vi "Configure DAQ (by ref).vi"(0 "System Ref":tag, 1 "Cal Files Path":path, 4 "Config":T3={"DAQ Settings"={"Trigger Type"=enum."Manual", "Trigger Samples"=0, "Pretrigger Samples"=0, "Trigger Interval"=0.0, "Time Units"=FALSE, "Auto Save"=FALSE, "Sample Rate"=7.0, "Select Analog"=FALSE, "Trigger Value"=0.0, "Trigger Stop Method"=enum."Use Samples Value to Stop Trigger", "Rate Sec/Min"=FALSE, "Save Mode"=enum."Single File", "File Size Limit"=0.0, "Log File Type"=enum."Basic", "Trigger Data Index"=0, "Log Rate"=7.0, "Rate Sec/Min (Log)"=FALSE, "Sample Rate (S/s)"=0.0, "Log Rate (S/s)"=0.0}, "Channels"=[], "Header"={"CA Number"="", "Test Name"="", "Serial Number"="", "Technician"=""}, "Graph Settings"={"Graph Labels"=[], [], [], [], [], [], [], [], [], [], [], [], [], "Graph Toggles"=[], "Axis Toggles"=[], "Graph Range"=enum."1"}, "Test Limits"=[], "All Type Info"=[], "Save Mode"=enum."Single File", "Data Base Path"=path ""} {"DAQ Settings"."Trigger Interval" min=0.0; "DAQ Settings"."Pretrigger Samples" min=0; "DAQ Settings"."Trigger Samples" min=0}, 5 "Channel Filter":bool[](array[boolean])=[FALSE, TRUE, TRUE, TRUE, TRUE, TRUE, TRUE, TRUE, TRUE, TRUE, TRUE, TRUE, TRUE, TRUE, TRUE, TRUE, TRUE, TRUE, TRUE, TRUE, TRUE, TRUE, TRUE, TRUE, TRUE, TRUE, TRUE, TRUE, TRUE, TRUE, TRUE, TRUE, TRUE, TRUE, TRUE, TRUE, TRUE, TRUE, TRUE, TRUE, TRUE, TRUE, TRUE, TRUE, TRUE, TRUE, TRUE, TRUE, TRUE], 7 "Sensor (scaling)":T2(array[cluster]), 8 "Manual/Timed Trigger":bool, 9 "Mode":enum16{"Init", "Acquire", "Clear"}(ring), 11 "System Type":T1, 14 "Total Channel Count":i16, 15 "Time Offset":dbl) -> (16 "Pretrigger Size":i32, 20 "Input Task OUT":refnum<k21>, 21 "Acquiring Data":bool, 22 "Ctr Task OUT":refnum<k21>, 24 "DAQ Complete Trigger":bool, 25 "Data":sgl[][](array[numeric]), 26 "DI Task OUT":refnum<k21>, 27 "error out":errorcluster={"status"=TRUE, "code"=-10621, "source"="AI Control"})   [LabVIEW 2023]
uses:
  Type Defs and Controls/Sensor Config.ctl
  Type Defs and Controls/DAQ Settings.ctl
  Type Defs and Controls/Trigger Stop Method.ctl
  Type Defs and Controls/Log File Type.ctl
  Type Defs and Controls/Channel Config.ctl
  Type Defs and Controls/Header.ctl
  Type Defs and Controls/Graph Settings Type Def.ctl
  Type Defs and Controls/Test Limits.ctl
  Type Defs and Controls/All Part Info.ctl
  Type Defs and Controls/Part Info.ctl
  Type Defs and Controls/System Type.ctl
  Type Defs and Controls/Coeffs Cluster Type Def.ctl
  <vilib>/DAQmx/read.llb/DAQmx Read (Counter 1D DBL 1Chan NSamp).vi
  <vilib>/DAQmx/read.llb/DAQmx Read (Analog 2D DBL NChan NSamp).vi
  <vilib>/DAQmx/miscellaneous.llb/DAQmx Fill In Error Info.vi
  <vilib>/measure/mamon.llb/Trigger Detection for 1 Channel (obs).vi
  <vilib>/measure/NI_MAPro.lvlib
  <resource>/objmgr/daqmx.rc
panel:
  out "Acquiring Data":bool
  # "EGU"
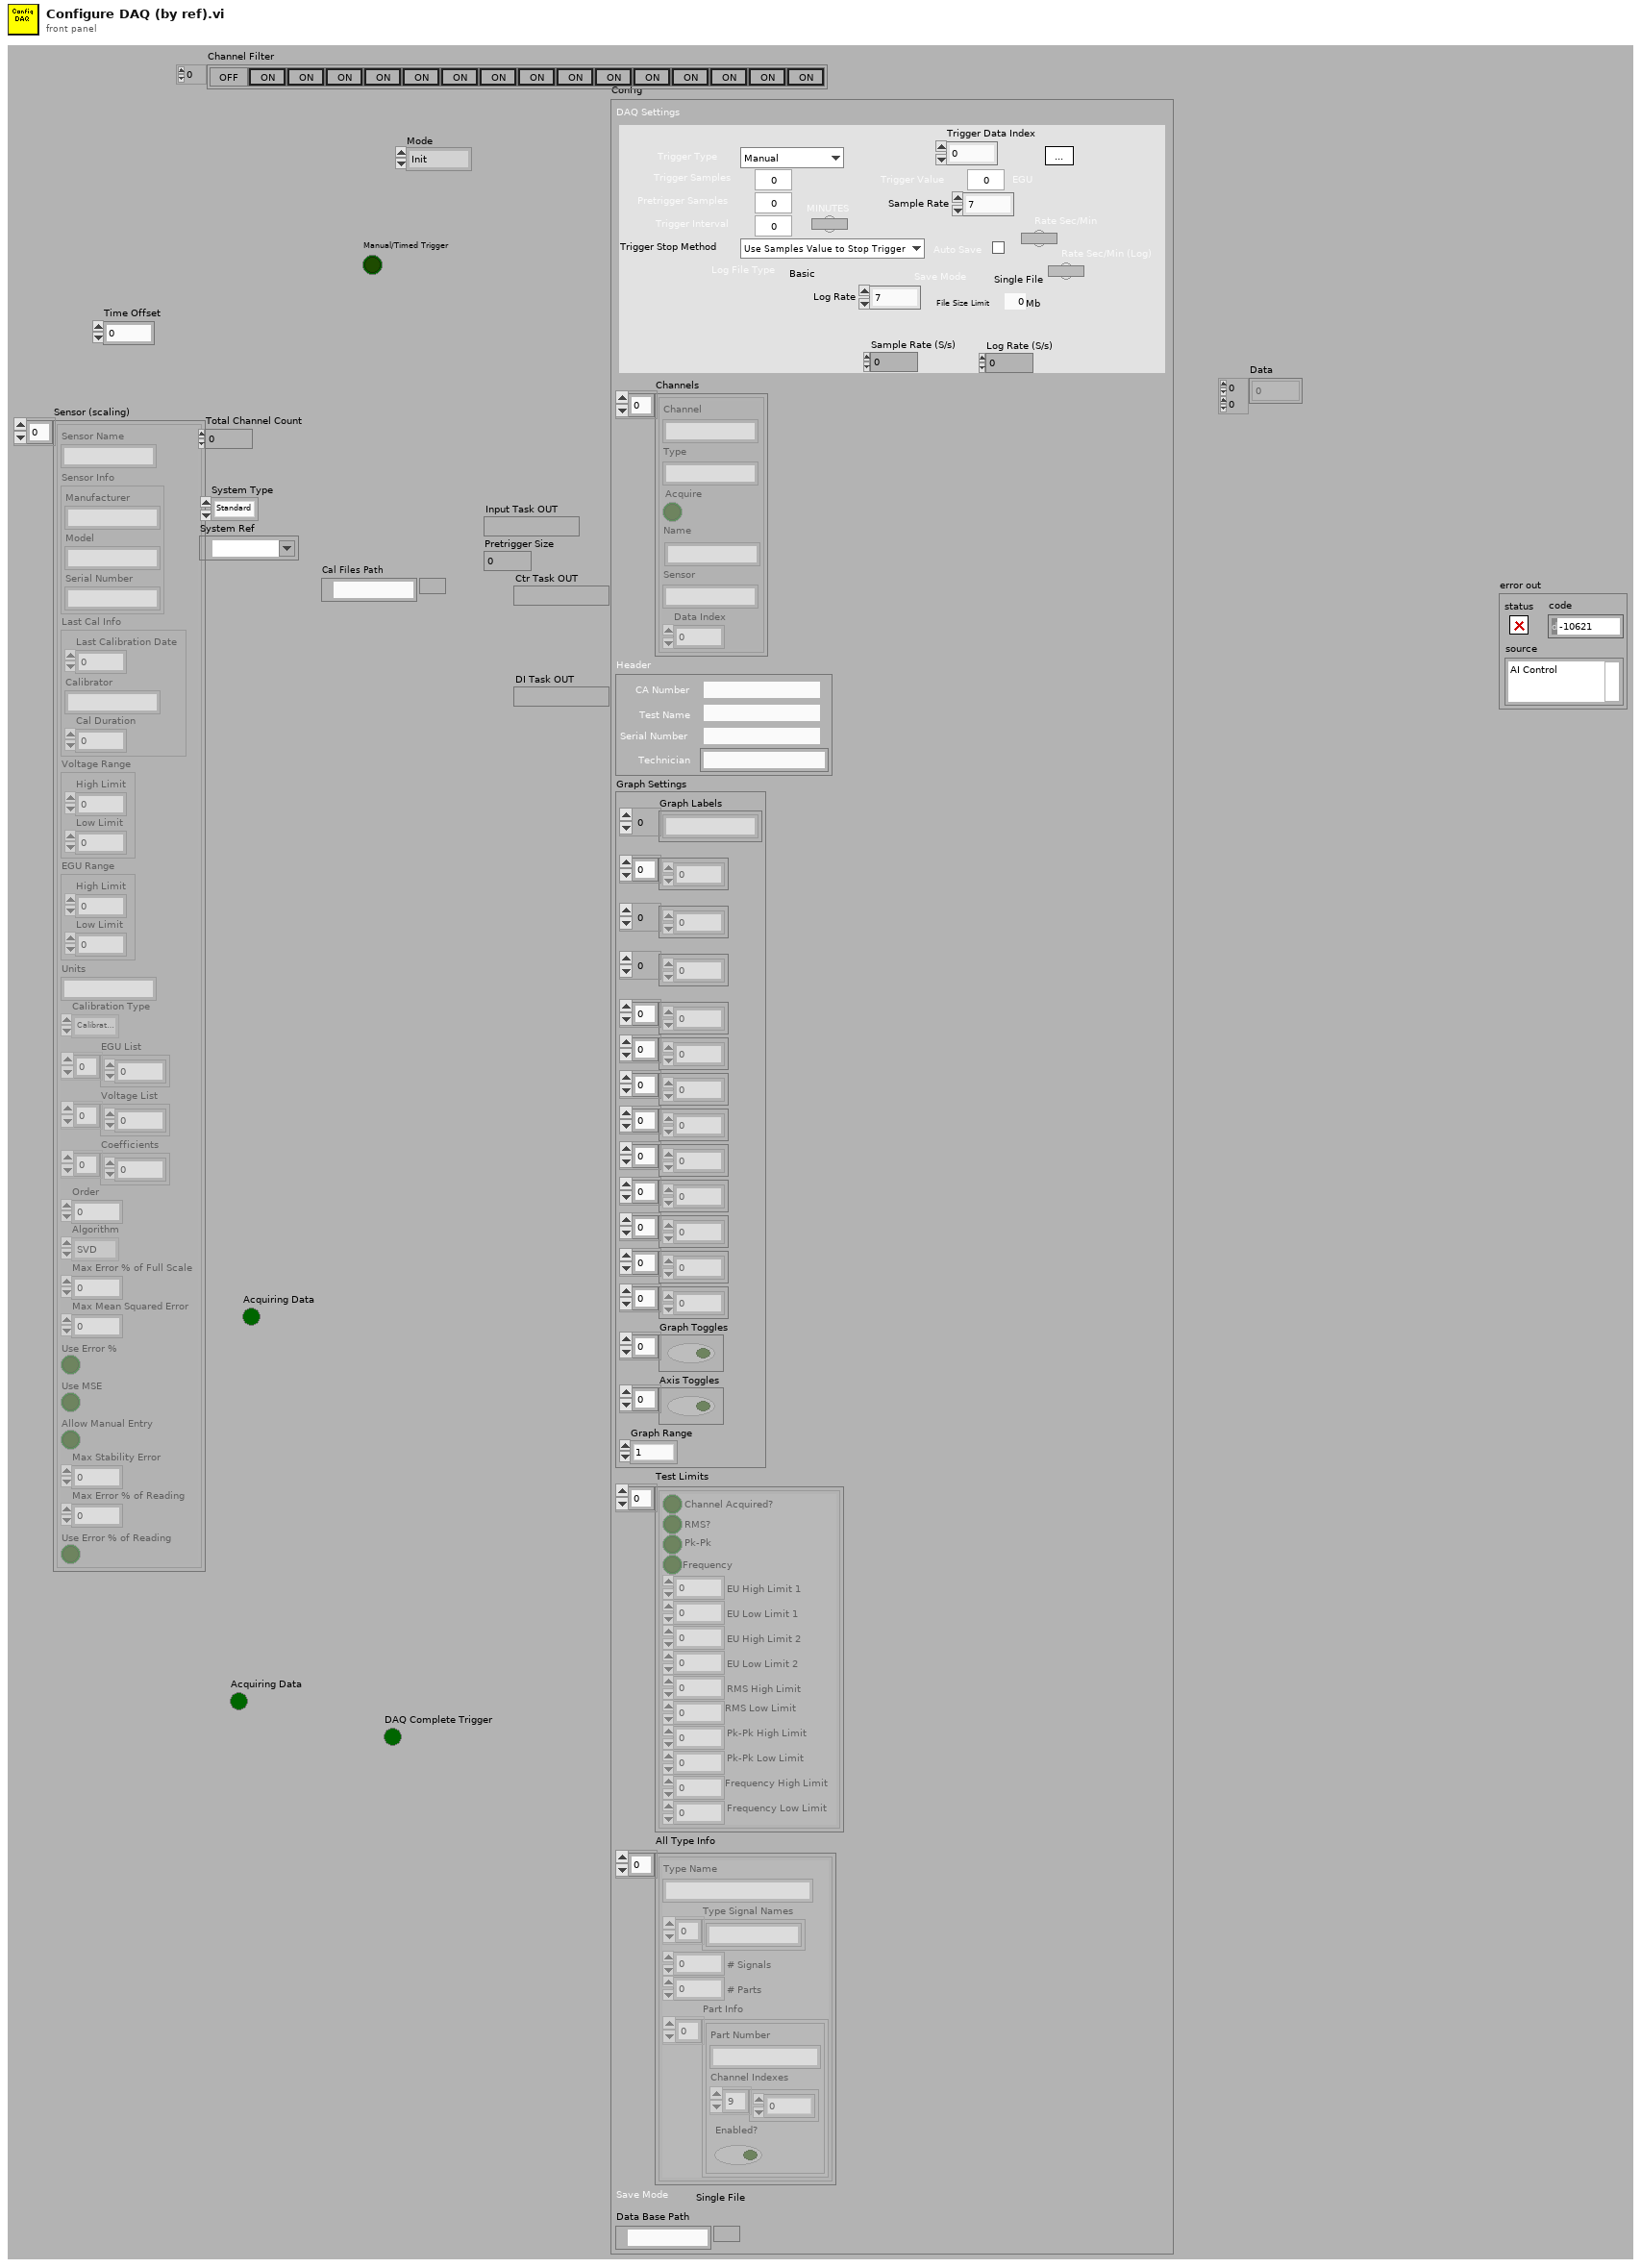
[diagram p1: front panel]
types:
  T1 = typedef "System Type.ctl" = enum16{"Standard", "Deformation", "Standard 8TC"}
  T2 = cluster{"Sensor Name":string, "Sensor Info":cluster{"Manufacturer":string, "Model":string, "Serial Number":string}, "Last Cal Info":cluster{"Last Calibration Date":dbl, "Calibrator":string, "Cal Duration":i32}, "Voltage Range":cluster{"High Limit":dbl, "Low Limit":dbl}, "EGU Range":cluster{"High Limit":dbl, "Low Limit":dbl}, "Units":string, "Calibration Type":enum16{"Calibrate Analog", "Compare Analog Calibration"}, "EGU List":dbl[], "Voltage List":dbl[], "Coefficients":dbl[], "Order":i32, "Algorithm":enum32{"SVD", "Givens", "Givens2", "Householder", "LU Decomposition", "Cholesky"}, "Max Error % of Full Scale":dbl, "Max Mean Squared Error":dbl, "Use Error %":bool, "Use MSE":bool, "Allow Manual Entry":bool, "Max Stability Error":dbl, "Max Error % of Reading":dbl, "Use Error % of Reading":bool}[]
  T3 = typedef "Sensor Config.ctl" = cluster{"DAQ Settings":T4, "Channels":T7[], "Header":T8, "Graph Settings":T9, "Test Limits":T10[], "All Type Info":T11, "Save Mode":enum16{"Single File", "Segmented Files", "New File at Midnight"}, "Data Base Path":path}
  T4 = typedef "DAQ Settings.ctl" = cluster{"Trigger Type":enum16{"Manual", "Timed", "Analog Rising", "Analog Falling"}, "Trigger Samples":i32, "Pretrigger Samples":i32, "Trigger Interval":dbl, "Time Units":bool, "Auto Save":bool, "Sample Rate":dbl, "Select Analog":bool, "Trigger Value":dbl, "Trigger Stop Method":T5, "Rate Sec/Min":bool, "Save Mode":enum16{"Single File", "Segmented Files", "New File at Midnight"}, "File Size Limit":dbl, "Log File Type":T6, "Trigger Data Index":u32, "Log Rate":dbl, "Rate Sec/Min (Log)":bool, "Sample Rate (S/s)":dbl, "Log Rate (S/s)":dbl}
  T5 = typedef "Trigger Stop Method.ctl" = enum16{"Use Samples Value to Stop Trigger", "Use Threshold to Stop Trigger"}
  T6 = typedef "Log File Type.ctl" = enum16{"Basic", "RTS"}
  T7 = typedef "Channel Config.ctl" = cluster{"Channel":string, "Type":string, "Acquire":bool, "Name":string, "Sensor":string, "Data Index":u32}
  T8 = typedef "Header.ctl" = cluster{"CA Number":string, "Test Name":string, "Serial Number":string, "Technician":string}
  T9 = typedef "Graph Settings Type Def.ctl" = cluster{"Graph Labels":string[], u8[], i16[], u32[], u8[], u8[], u8[], u32[], u8[], u8[], u8[], dbl[], dbl[], "Graph Toggles":bool[], "Axis Toggles":bool[], "Graph Range":enum16{"1", "2", "3", "4", "5", "10", "15", "30", "60"}}
  T10 = typedef "Test Limits.ctl" = cluster{"Channel Acquired?":bool, "RMS?":bool, "Pk-Pk":bool, "Frequency":bool, "EU High Limit 1":dbl, "EU Low Limit 1":dbl, "EU High Limit 2":dbl, "EU Low Limit 2":dbl, "RMS High Limit":dbl, "RMS Low Limit":dbl, "Pk-Pk High Limit ":dbl, "Pk-Pk Low Limit":dbl, "Frequency High Limit":dbl, "Frequency Low Limit":dbl}
  T11 = typedef "All Part Info.ctl" = cluster{"Type Name":string, "Type Signal Names":string[], "# Signals":i32, "# Parts":i32, "Part Info":T12[]}[]
  T12 = typedef "Part Info.ctl" = cluster{"Part Number":string, "Channel Indexes":u16[], "Enabled?":bool}
  T13 = typedef "Coeffs Cluster Type Def.ctl" = cluster{"AI Coeffs":cluster{"Coefficients":dbl[]}[]}
  T14 = cluster{"Coefficients":cluster{"Coefficients":dbl[]}[]}
  T15 = enum16{"Manual", "Timed", "Analog Rising", "Analog Falling"}
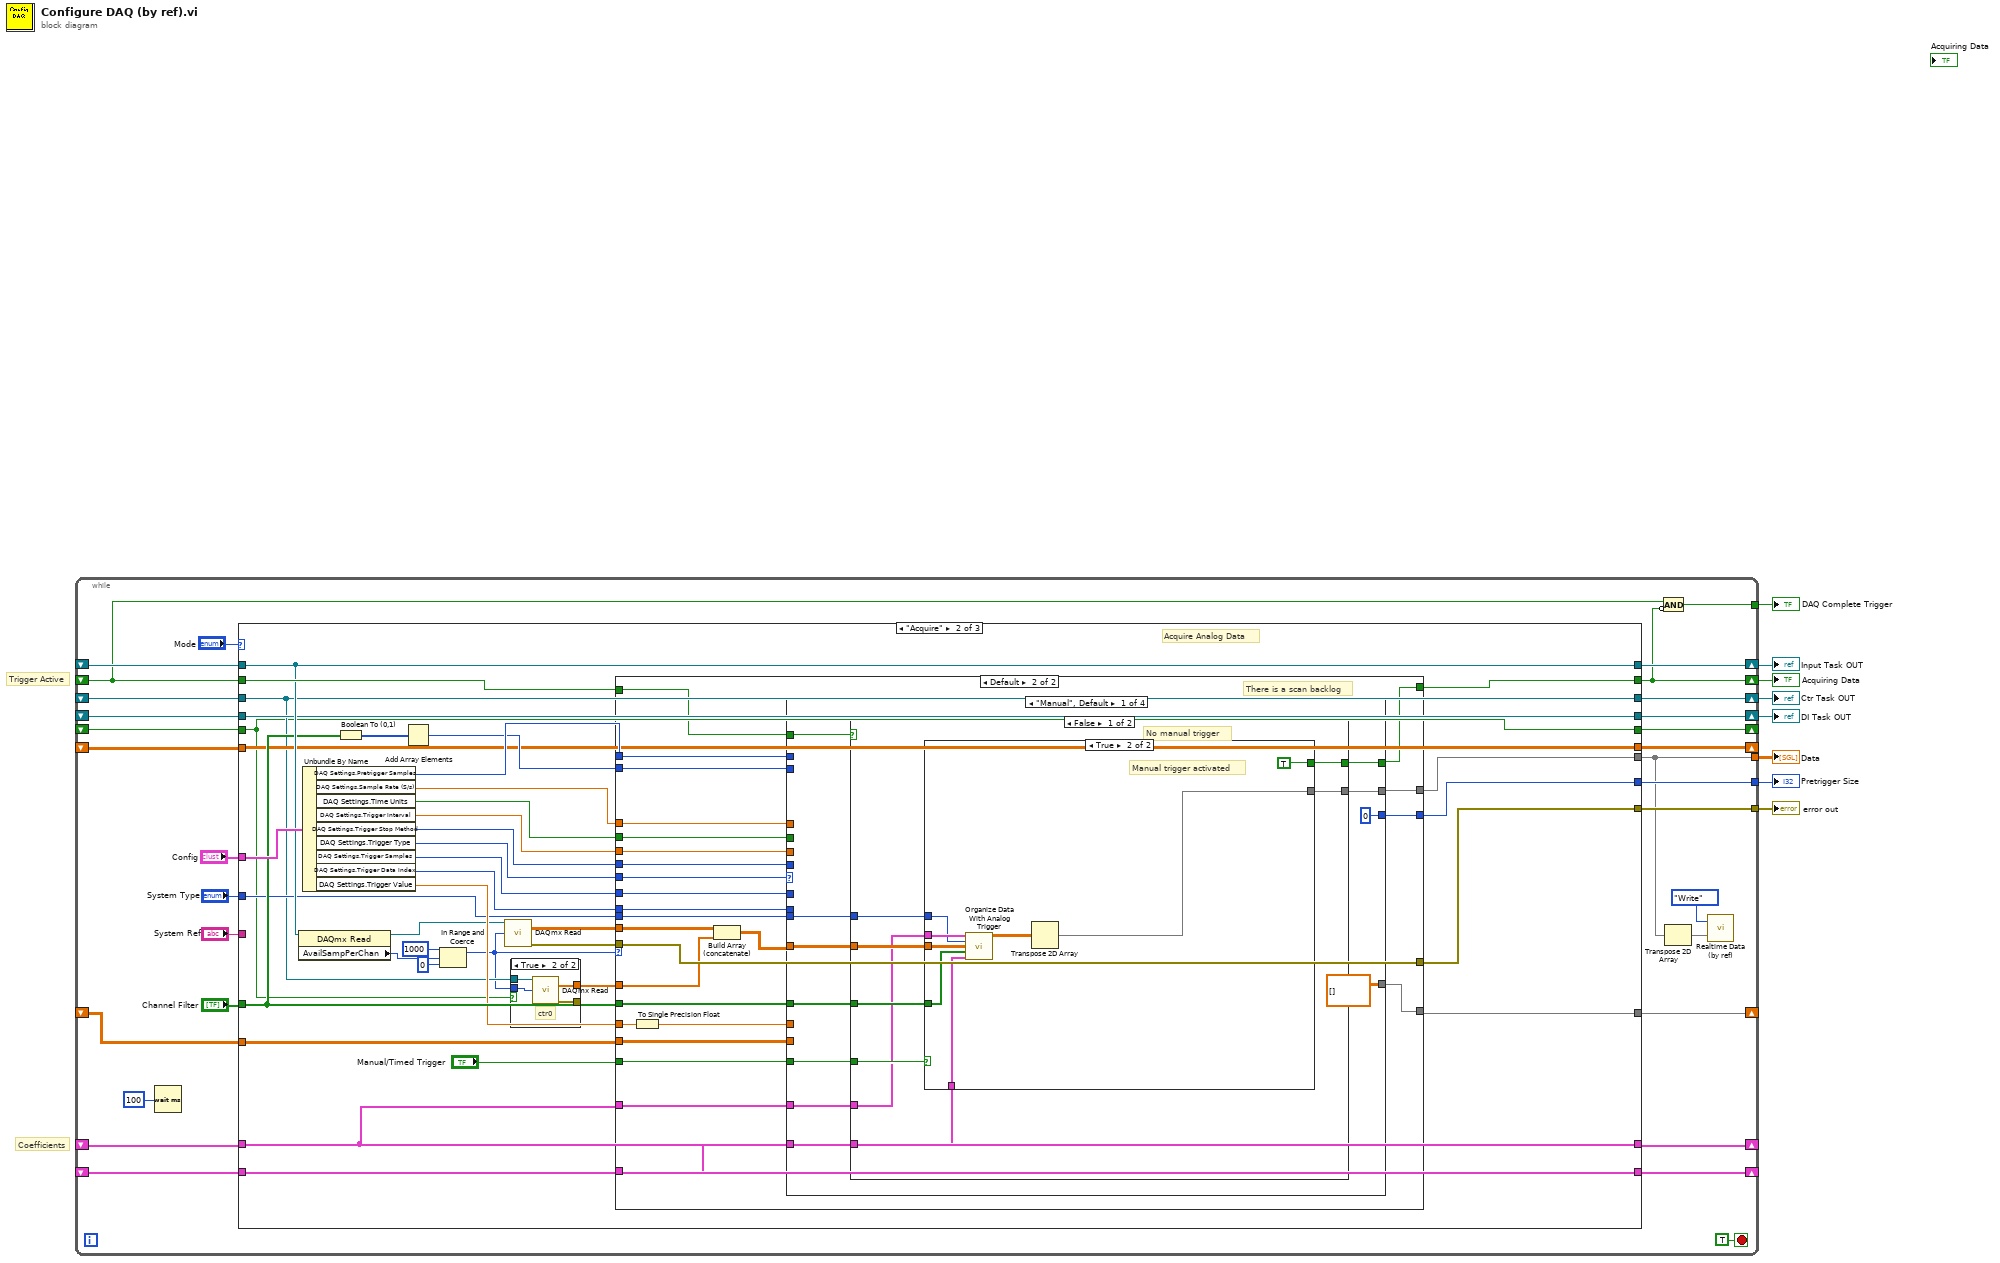
[diagram p0: block diagram]
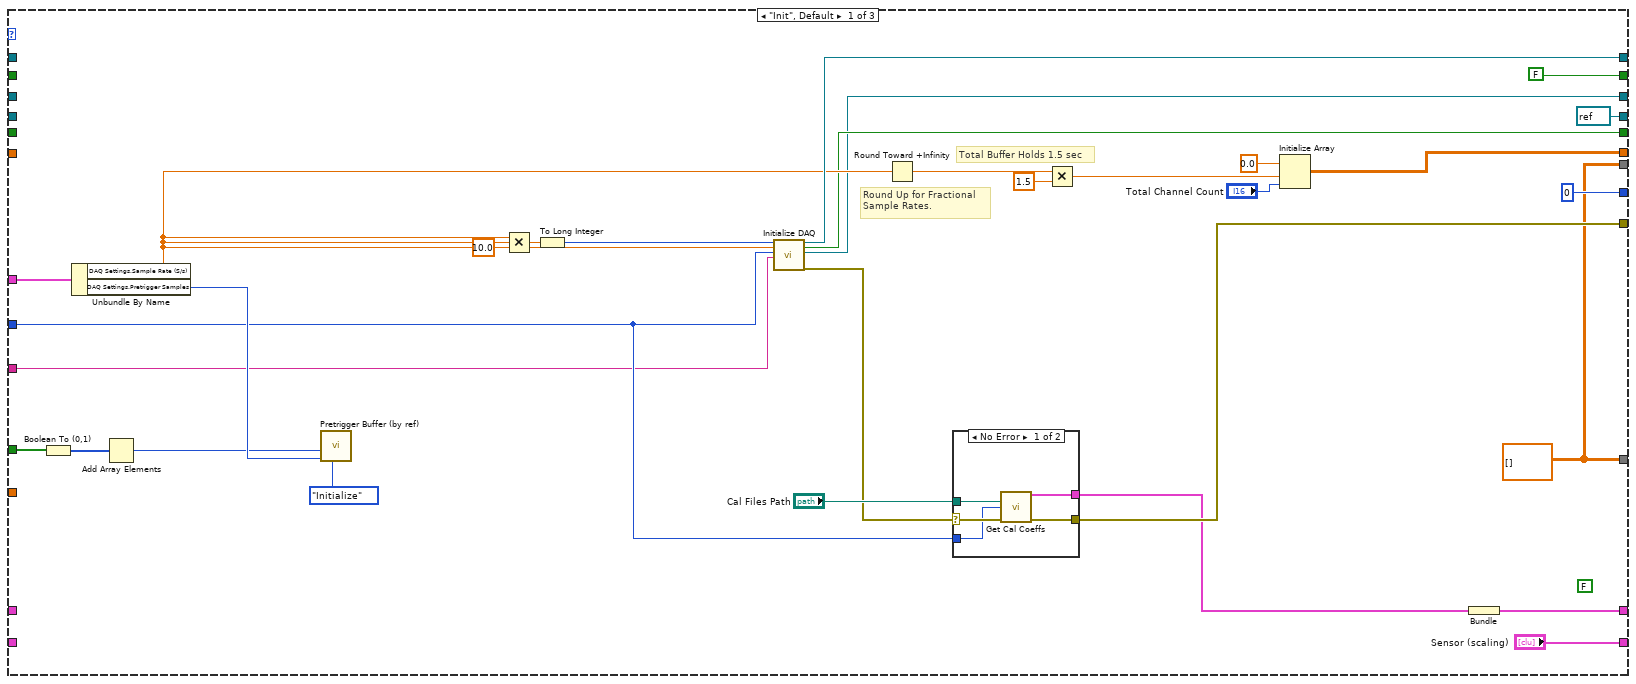
[diagram p2: hidden frame]
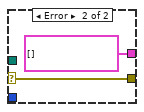
[diagram p3: hidden frame]
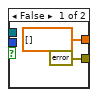
[diagram p4: hidden frame]
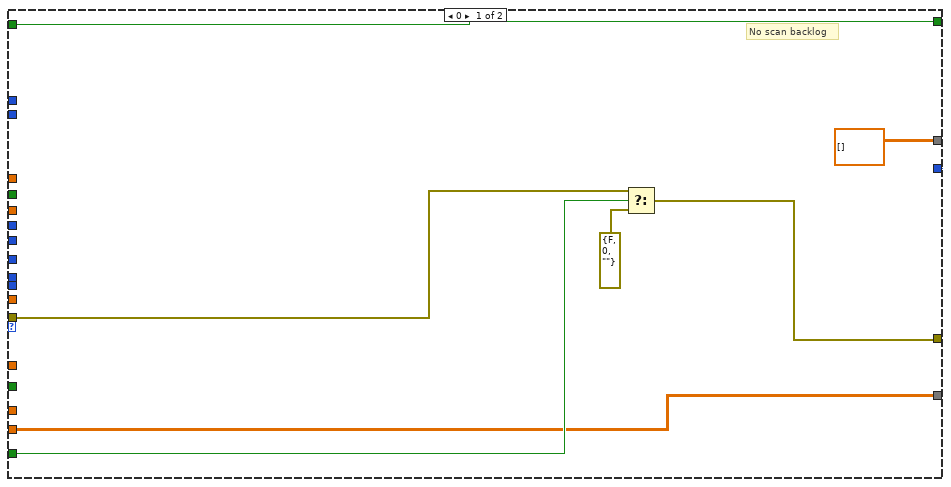
[diagram p5: hidden frame]
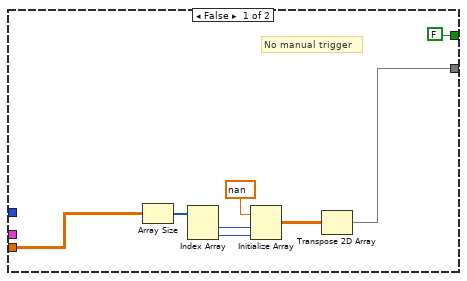
[diagram p6: hidden frame]
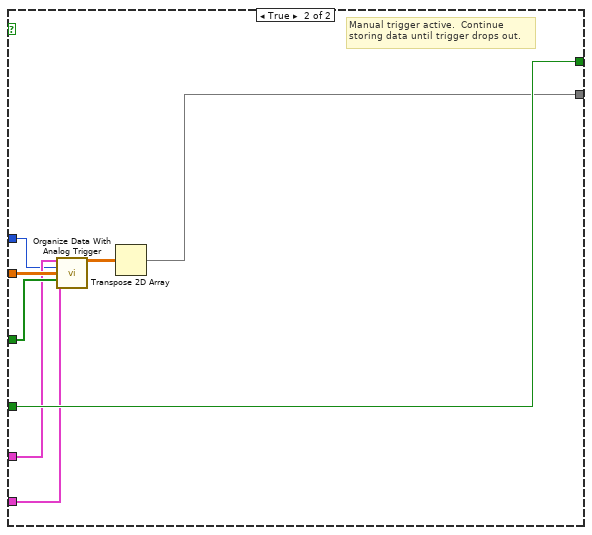
[diagram p7: hidden frame]
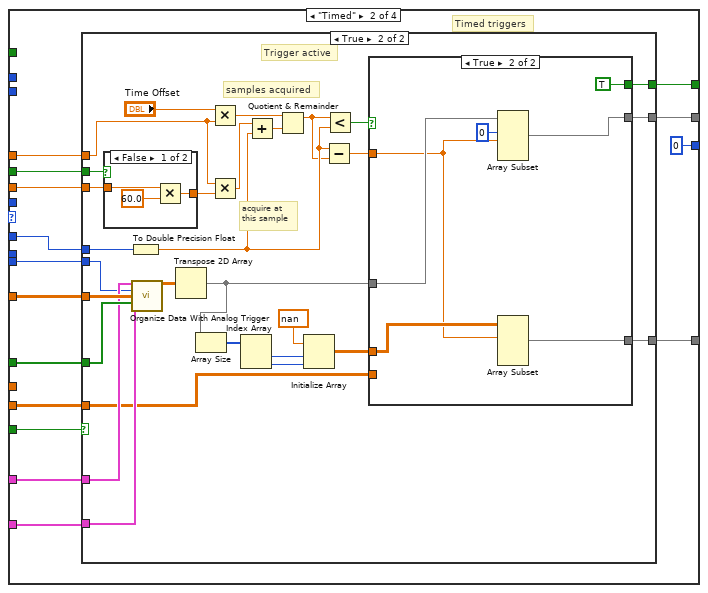
[diagram p8: hidden frame]
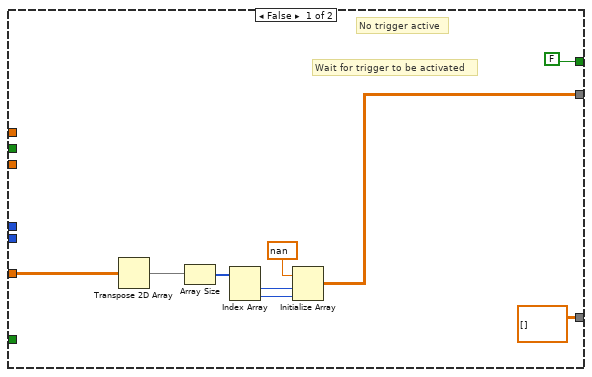
[diagram p9: hidden frame]
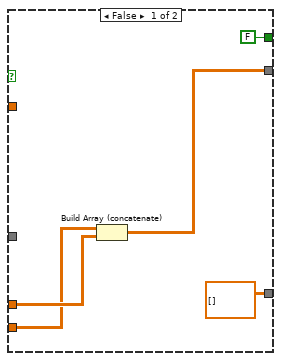
[diagram p10: hidden frame]
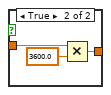
[diagram p11: hidden frame]
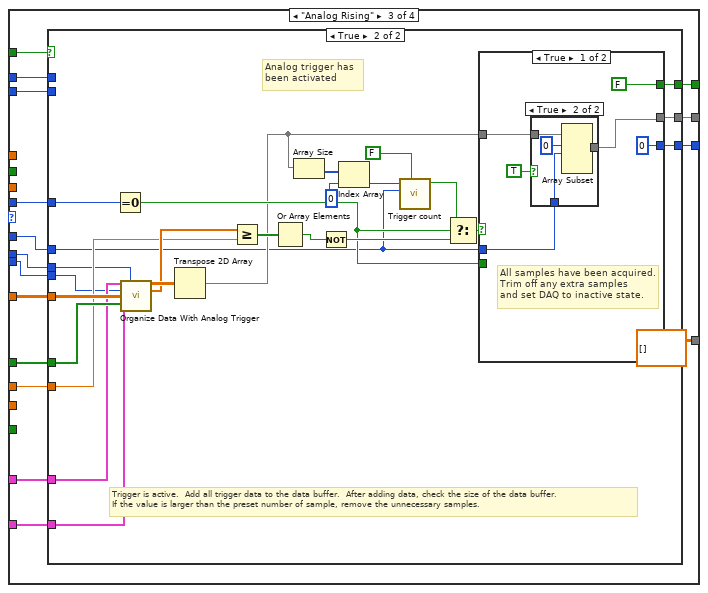
[diagram p12: hidden frame]
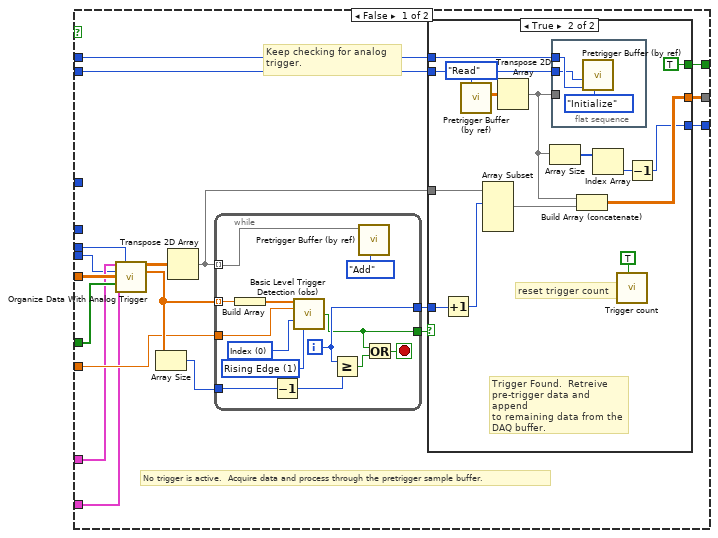
[diagram p13: hidden frame]
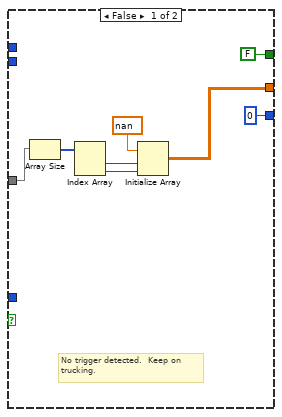
[diagram p14: hidden frame]
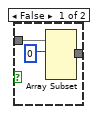
[diagram p15: hidden frame]
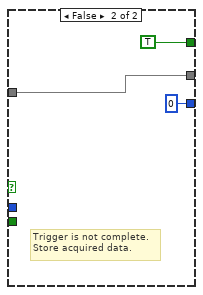
[diagram p16: hidden frame]
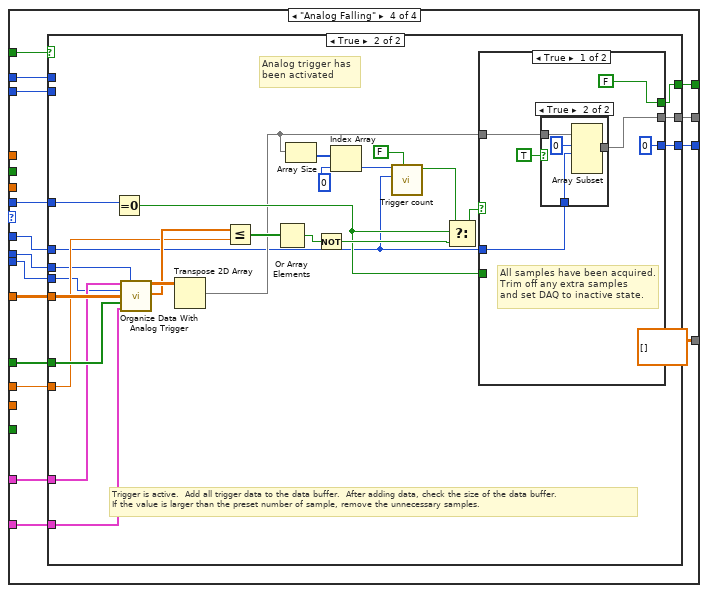
[diagram p17: hidden frame]
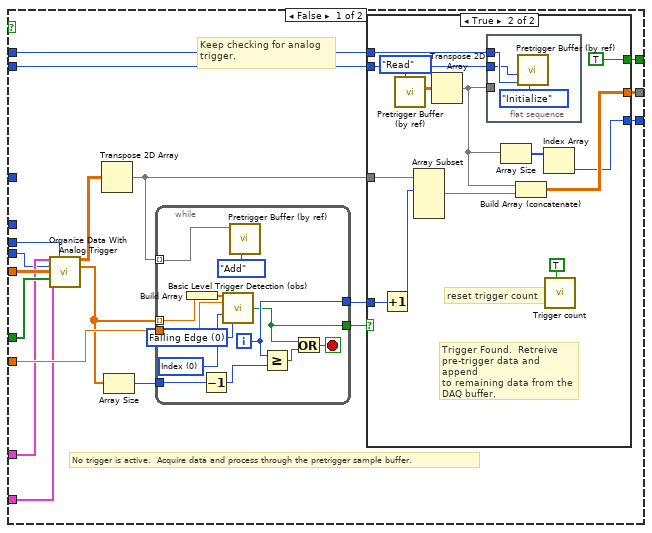
[diagram p18: hidden frame]
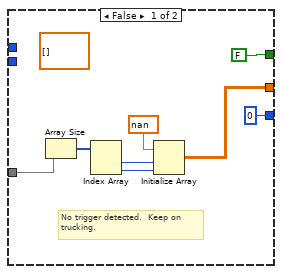
[diagram p19: hidden frame]
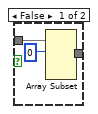
[diagram p20: hidden frame]
diagram:
  # "Coefficients"
  # "Trigger Active"
  n1 = while {
    shift-right: [w34] -> w5
    shift-left: _ -> [w36]
    tunnel: [w37] -> w8
    shift-right: [w32] -> w7
    shift-left: _ -> [w30]
    tunnel: [w31] -> w6
    shift-right: [w29] -> _
    shift-left: _ -> [w28]
    shift-right: [w24] -> _
    shift-left: _ -> [w25]
    tunnel: [w23] -> w4
    shift-right: [w22] -> _
    shift-left: _ -> [w21]
    shift-right: [w18] -> _
    shift-left: _ -> [w19]
    tunnel: [w17] -> w3
    shift-right: [w16] -> w2
    shift-left: _ -> [w15]
    shift-right: [w14] -> w1
    shift-left: _ -> [w13]
    shift-right: [w11] -> _
    shift-left: _ -> [w10]
    stop <- TRUE stop-if-true
    n2 = Wait (ms)(milliseconds to wait=u32 100) -> ()  [unwired: 1 out]
    n3 = case shown="\"Acquire\"" "Mode" {
      tunnel: [w56 w91 errorcluster {"status"=FALSE, "code"=0, "source"=""} ("error out")] -> w37
      tunnel: w36 -> [_ w104 w505]
      tunnel: "Config" -> [w68 w108 _]
      tunnel: [w60 w104 refnum<k21> refnum ("task out")] -> w34
      tunnel: [FALSE w112 FALSE] -> w32
      tunnel: w30 -> [_ w110 _]
      tunnel: [w48 w88 w501] -> w17
      tunnel: "Channel Filter" -> [w58 w101 _]
      tunnel: ["Sensor (scaling)" w107 w507] -> w29
      tunnel: w28 -> [_ w107 w507]
      tunnel: [w45 w93 T13 {"AI Coeffs"=[]} ("Coefficients")] -> w24
      tunnel: w25 -> [_ w93 _]
      tunnel: [0 w99 0] -> w23
      tunnel: [w48 w96 w501] -> w22
      tunnel: w21 -> [_ w95 _]
      tunnel: w19 -> [_ w89 w502]
      tunnel: [w49 w89 w502] -> w18
      tunnel: [w41 w80 refnum<k21> refnum ("DO Task OUT")] -> w16
      tunnel: w15 -> [_ w80 w499]
      tunnel: [refnum<k21> refnum ("DO Task OUT") w92 refnum<k21> refnum ("DO Task OUT")] -> w14
      tunnel: w13 -> [_ w92 w497]
      tunnel: "System Type" -> [w43 w81 _]
      tunnel: [w42 w78 FALSE ("Ctr Present")] -> w11
      tunnel: w10 -> [_ w78 _]
      tunnel: "System Ref" -> [w40 _ _]
      frame "Init", Default {
        (unwired) FALSE ("data")
        w48 = sgl[][] []
        # "Round Up for Fractional\nSample Rates."
        # "Total Buffer Holds 1.5 sec"
        n4 = Boolean To (0,1)(Boolean=w58) -> (0, 1=w64:i16[])
        n5 = Unbundle By Name(w68) -> ("DAQ Settings.Sample Rate (S/s)"=w53:dbl, "DAQ Settings.Pretrigger Samples"=w65:i32)
        n6 = Add Array Elements(numeric array=w64) -> (sum=w63:i16)
        n7 = call "Pretrigger Buffer (by ref).vi"("Mode"=enum16{"Initialize", "Add", "Read"}."Initialize", "Pretrigger Length"=w65, "# Channels"=w63) -> ()  [unwired: 6 in, 2 out]
        n8 = Multiply(x=w53, y=sgl 10.0) -> ()  [unwired: 1 out]
        n9 = To Long Integer(number=w53) -> (32bit integer=w61:i32)
        n10 = call "Initialize DAQ.vi"("number of samples"=w61, "rate"=w53, "System Type"=w43, "System Ref"=w40) -> ("AI Task OUT"=w60:refnum<k21>, "Ctr Present"=w42:bool, "Ctr Task OUT"=w41:refnum<k21>, "error out"=w57:errorcluster)  [unwired: 12 in]
        n11 = Round Toward +Infinity(x=w53) -> (ceil(x): smallest int >= x=w47:dbl)
        n12 = case shown="No Error" w57 {
          selector: w57 -> [w72 w76]
          tunnel: "Cal Files Path" -> [w74 _]
          tunnel: [w73 cluster{"Coefficients":dbl[]}[] [] ("Coefficients")] -> w46
          tunnel: [w71 w76] -> w56
          tunnel: w43 -> [w70 _]
          frame No Error {
            n13 = call "Get Cal Coeffs.vi"("Cal Files Path"=w74, "System Type"=w70, "Error IN"=w72) -> ("AI Coeffs"=w73:cluster{"Coefficients":dbl[]}[], "Error OUT"=w71:errorcluster)  [unwired: 11 in]
          }
          frame Error {
          }
        }
        n14 = Multiply(x=w47, y=1.5) -> (x*y=w50:dbl)
        n15 = Initialize Array(sgl 0.0 ("element"), w50, "Total Channel Count") -> (w49:sgl[][])
        n16 = Bundle("Coefficients"=w46) -> (w45:T14)  [unwired: 1 in]
      }
      frame "Acquire" {
        # "Acquire Analog Data"
        n17 = property class="DAQmx Read"(reference=w104) -> (reference out=w84:refnum<k21>, "AvailSampPerChan"=w85:u32)  [unwired: 1 in, 1 out]
        n18 = Unbundle By Name(w108) -> ("DAQ Settings.Pretrigger Samples"=w103:i32, "DAQ Settings.Sample Rate (S/s)"=w97:dbl, "DAQ Settings.Time Units"=w98:bool, "DAQ Settings.Trigger Interval"=w105:dbl, "DAQ Settings.Trigger Stop Method"=w106:T5, "DAQ Settings.Trigger Type"=w113:T15, "DAQ Settings.Trigger Samples"=w111:i32, "DAQ Settings.Trigger Data Index"=w94:u32, "DAQ Settings.Trigger Value"=w90:dbl)
        n19 = Boolean To (0,1)(Boolean=w101) -> (0, 1=w102:i16[])
        n20 = Add Array Elements(numeric array=w102) -> (sum=w100:i16)
        n21 = In Range and Coerce(upper limit=u32 1000, x=w85, lower limit=u32 0) -> (coerced(x)=w79:u32)  [unwired: 1 out]
        n22 = call-poly <vilib>:"DAQmx Read.vi"("task/channels in"=w84, "number of samples per channel"=w79) -> ("data"=w82:dbl[][], "error out"=w83:errorcluster)  [unwired: 11 in, 1 out]
        n23 = case shown="True" w78 {
          tunnel: w80 -> [_ w119]
          tunnel: w79 -> [_ w118]
          tunnel: [dbl[] [] ("data") w117] -> w77
          tunnel: [errorcluster {"status"=FALSE, "code"=0, "source"=""} ("error out") w116] -> _
          frame False {
          }
          frame True {
            # "ctr0"
            n24 = call-poly <vilib>:"DAQmx Read.vi"("task/channels in"=w119, "number of samples per channel"=w118) -> ("data"=w117:dbl[], "error out"=w116:errorcluster)  [unwired: 11 in, 1 out]
          }
        }
        n25 = case shown="Default" w79 {
          tunnel: w113 -> [_ w153]
          tunnel: w90 -> [_ w152]
          tunnel: [w127 w150] -> w112
          tunnel: w101 -> [_ w149]
          tunnel: w111 -> [_ w148]
          tunnel: w110 -> [w127 w133]
          tunnel: "Manual/Timed Trigger" -> [w125 w147]
          tunnel: w107 -> [_ w146]
          tunnel: w106 -> [_ w145]
          tunnel: w105 -> [_ w144]
          tunnel: w93 -> [_ w143]
          tunnel: [w126 w132] -> w91
          tunnel: w103 -> [_ w142]
          tunnel: w100 -> [_ w141]
          tunnel: [0 w140] -> w99
          tunnel: w98 -> [_ w139]
          tunnel: w97 -> [_ w138]
          tunnel: [w122 w137] -> w96
          tunnel: w95 -> [w122 w136]
          tunnel: w94 -> [_ w135]
          tunnel: [sgl[][] [] ("Scaled Data") w134] -> w88
          tunnel: w83 -> [w120 w132]
          tunnel: w82 -> [_ w130]
          tunnel: w81 -> [_ w131]
          tunnel: w77 -> [_ w129]
          frame 0 {
            # "No scan backlog"
            n26 = Select(t=w120, s=w125, f=errorcluster {"status"=FALSE, "code"=0, "source"=""} ("t")) -> (s? t:f=w126:errorcluster)
          }
          frame Default {
            # "There is a scan backlog"
            n27 = To Single Precision Float(number=w152) -> (single precision float=w151:sgl)
            n28 = Build Array (concatenate)(w130, w129) -> (w128:dbl[][])
            n29 = case shown="\"Manual\", Default" w153 {
              tunnel: w133 -> [w163 _ w283 w397]
              tunnel: w128 -> [w162 w210 w282 w396]
              tunnel: w151 -> [_ _ w281 w395]
              tunnel: [w159 w208 w280 w394] -> w150
              tunnel: [w164 w211 w279 w393] -> w134
              tunnel: w149 -> [w160 w209 w278 w392]
              tunnel: w148 -> [_ w207 w277 w391]
              tunnel: w147 -> [w161 w198 _ _]
              tunnel: w146 -> [w158 w206 w276 w390]
              tunnel: w145 -> [_ _ w275 w389]
              tunnel: w144 -> [_ w205 _ _]
              tunnel: w143 -> [w157 w204 w274 w388]
              tunnel: w142 -> [_ _ w273 w387]
              tunnel: w141 -> [_ _ w272 w386]
              tunnel: [0 0 w271 w385] -> w140
              tunnel: w139 -> [_ w202 _ _]
              tunnel: w138 -> [_ w201 _ _]
              tunnel: [sgl[][] [] w200 sgl[][] [] sgl[][] []] -> w137
              tunnel: w136 -> [_ w199 _ _]
              tunnel: w135 -> [_ _ w269 w383]
              tunnel: w131 -> [w154 w197 w268 w382]
              frame "Manual", Default {
                n30 = case shown="False" w163 {
                  tunnel: [w171 w191] -> w164
                  tunnel: w162 -> [w170 w196]
                  tunnel: w161 -> [w172 w195]
                  tunnel: w160 -> [w169 w193]
                  tunnel: [w168 w195] -> w159
                  tunnel: w158 -> [w167 w192]
                  tunnel: w157 -> [w166 w190]
                  tunnel: w154 -> [w165 w189]
                  frame False {
                    # "No manual trigger"
                    n31 = case shown="True" w172 {
                      tunnel: [w173 w183] -> w171
                      tunnel: w170 -> [w175 w188]
                      tunnel: w169 -> [_ w186]
                      tunnel: [FALSE TRUE] -> w168
                      tunnel: w167 -> [_ w185]
                      tunnel: w166 -> [_ w182]
                      tunnel: w165 -> [_ w181]
                      frame False {
                        # "No manual trigger"
                        n32 = Array Size(array=w175) -> (size(s)=w179:i32[])
                        n33 = Index Array(array=w179) -> (element #1=w178:i32, element #2=w177:i32)  [unwired: 2 in]
                        n34 = Initialize Array(sgl nan ("element"), w178, w177) -> (w174:sgl[][])
                        n35 = Transpose 2D Array(2D array=w174) -> (transposed array=w173:sgl[][])
                      }
                      frame True {
                        # "Manual trigger activated"
                        n36 = call "Organize Data With Analog Trigger.vi"("Coefficients"=w182, "System Type"=w181, "DAQ"=w188, "Channel Filter"=w186, "Sensor (scaling)"=w185) -> ("Scaled Data"=w184:sgl[][])  [unwired: 9 in, 1 out]
                        n37 = Transpose 2D Array(2D array=w184) -> (transposed array=w183:sgl[][])
                      }
                    }
                  }
                  frame True {
                    # "Manual trigger active.  Continue\nstoring data until trigger drops out."
                    n38 = call "Organize Data With Analog Trigger.vi"("Coefficients"=w190, "System Type"=w189, "DAQ"=w196, "Channel Filter"=w193, "Sensor (scaling)"=w192) -> ("Scaled Data"=w194:sgl[][])  [unwired: 9 in, 1 out]
                    n39 = Transpose 2D Array(2D array=w194) -> (transposed array=w191:sgl[][])
                  }
                }
              }
              frame "Timed" {
                # "Timed triggers"
                n40 = case shown="True" w198 {
                  tunnel: [w220 w235] -> w211
                  tunnel: w210 -> [w219 w249]
                  tunnel: w209 -> [_ w247]
                  tunnel: [FALSE w236] -> w208
                  tunnel: w207 -> [_ w239]
                  tunnel: w206 -> [_ w246]
                  tunnel: w205 -> [_ w243]
                  tunnel: w204 -> [_ w245]
                  tunnel: w202 -> [_ w244]
                  tunnel: w201 -> [_ w240]
                  tunnel: [sgl[][] [] w228] -> w200
                  tunnel: w199 -> [_ w227]
                  tunnel: w197 -> [_ w221]
                  frame False {
                    # "Wait for trigger to be activated"
                    # "No trigger active"
                    n41 = Transpose 2D Array(2D array=w219) -> (transposed array=w212:dbl[][])
                    n42 = Array Size(array=w212) -> (size(s)=w216:i32[])
                    n43 = Index Array(array=w216) -> (element #1=w213:i32, element #2=w215:i32)  [unwired: 2 in]
                    n44 = Initialize Array(sgl nan ("element"), w213, w215) -> (w220:sgl[][])
                  }
                  frame True {
                    # "acquire at\nthis sample"
                    # "samples acquired"
                    # "Trigger active"
                    n45 = case shown="False" w244 {
                      tunnel: w243 -> [w264 w266]
                      tunnel: [w262 w265] -> w241
                      frame False {
                        n46 = Multiply(x=w264, y=60.0) -> (x*y=w262:dbl)
                      }
                      frame True {
                        n47 = Multiply(x=w266, y=3600.0) -> (x*y=w265:dbl)
                      }
                    }
                    n48 = To Double Precision Float(number=w239) -> (double precision float=w224:dbl)
                    n49 = call "Organize Data With Analog Trigger.vi"("Coefficients"=w245, "System Type"=w221, "DAQ"=w249, "Channel Filter"=w247, "Sensor (scaling)"=w246) -> ("Scaled Data"=w248:sgl[][])  [unwired: 9 in, 1 out]
                    n50 = Transpose 2D Array(2D array=w248) -> (transposed array=w230:sgl[][])
                    n51 = Array Size(array=w230) -> (size(s)=w234:i32[])
                    n52 = Multiply(x="Time Offset", y=w240) -> (x*y=w226:dbl)
                    n53 = Multiply(x=w240, y=w241) -> (x*y=w225:dbl)
                    n54 = Index Array(array=w234) -> (element #1=w231:i32, element #2=w233:i32)  [unwired: 2 in]
                    n55 = Add(x=w225, y=w224) -> (x+y=w223:dbl)
                    n56 = Quotient & Remainder(x=w226, y=w223) -> (x-y*floor(x/y)=w222:dbl)  [unwired: 1 out]
                    n57 = Initialize Array(sgl nan ("element"), w231, w233) -> (w229:sgl[][])
                    n58 = Subtract(x=w224, y=w222) -> (x-y=w237:dbl)
                    n59 = Less?(x=w222, y=w224) -> (x < y?=w238:bool)
                    n60 = case shown="True" w238 {
                      tunnel: w237 -> [_ w257]
                      tunnel: w230 -> [_ w260]
                      tunnel: [FALSE TRUE] -> w236
                      tunnel: [w250 w256] -> w235
                      tunnel: w229 -> [w252 w258]
                      tunnel: [sgl[][] [] w255] -> w228
                      tunnel: w227 -> [w251 _]
                      frame False {
                        n61 = Build Array (concatenate)(w251, w252) -> (w250:sgl[][])
                      }
                      frame True {
                        n62 = Array Subset(array=w260, index (row)=0 ("index"), length (row)=w257) -> (w256:sgl[][])  [unwired: 2 in]
                        n63 = Array Subset(array=w258, index (row)=w257) -> (w255:sgl[][])  [unwired: 3 in]
                      }
                    }
                  }
                }
              }
              frame "Analog Rising" {
                n64 = case shown="True" w283 {
                  tunnel: w282 -> [w301 w365]
                  tunnel: w281 -> [w296 w354]
                  tunnel: [w300 w361] -> w280
                  tunnel: [w299 w362] -> w279
                  tunnel: w278 -> [w292 w359]
                  tunnel: w277 -> [_ w346]
                  tunnel: w276 -> [w291 w358]
                  tunnel: w275 -> [_ w357]
                  tunnel: w274 -> [w289 w344]
                  tunnel: w273 -> [w288 _]
                  tunnel: w272 -> [w287 _]
                  tunnel: [w286 w343] -> w271
                  tunnel: w269 -> [w285 w342]
                  tunnel: w268 -> [w284 w341]
                  frame False {
                    # "Keep checking for analog\ntrigger."
                    # "No trigger is active.  Acquire data and process through the pretrigger sample buffer."
                    n65 = call "Organize Data With Analog Trigger.vi"("Coefficients"=w289, "Trigger Data Index"=w285, "System Type"=w284, "DAQ"=w301, "Channel Filter"=w292, "Sensor (scaling)"=w291) -> ("Scaled Data"=w293:sgl[][], "trigger data"=w298:sgl[])  [unwired: 8 in]
                    n66 = Array Size(array=w298) -> (size(s)=w297:i32)
                    n67 = Transpose 2D Array(2D array=w293) -> (transposed array=w290:sgl[][])
                    n68 = while {
                      tunnel: w298 -> [w310] mode=indexing
                      tunnel: w296 -> [w308]
                      tunnel: [w304] -> w294
                      tunnel: w297 -> [w312]
                      tunnel: [w311] -> w295
                      tunnel: w290 -> [w302] mode=indexing
                      i -> [w311]
                      stop <- w313 stop-if-true
                      w306 = u16 1 items=["Falling Edge", "Rising Edge"] ("slope")
                      w307 = u16 0 items=["Index", "Time"] ("mode")
                      n69 = Build Array(w310) -> (w309:sgl[])
                      n70 = Decrement(x=w312) -> (x-1=w314:i32)
                      n71 = call-poly <vilib>:"Basic Level Trigger Detection (obs).vi"("signal in"=w309, "level"=w308, "location mode"=w307, "trigger slope"=w306) -> ("trigger detected?"=w304:bool)  [unwired: 9 in, 2 out]
                      n72 = Greater Or Equal?(x=w311, y=w314) -> (x >= y?=w305:bool)
                      n73 = call "Pretrigger Buffer (by ref).vi"("Mode"=enum16{"Initialize", "Add", "Read"}."Add", "New Data"=w302) -> ()  [unwired: 7 in, 2 out]
                      n74 = Or(x=w304, y=w305) -> (x .or. y?=w313:bool)
                    }
                    n75 = case shown="True" w294 {
                      tunnel: [FALSE TRUE] -> w300
                      tunnel: w290 -> [w321 w336]
                      tunnel: [w317 w332] -> w299
                      tunnel: w295 -> [_ w325]
                      tunnel: w288 -> [_ w330]
                      tunnel: w287 -> [_ w329]
                      tunnel: [0 w323] -> w286
                      frame False {
                        # "No trigger detected.  Keep on\ntrucking."
                        n76 = Array Size(array=w321) -> (size(s)=w320:i32[])
                        n77 = Index Array(array=w320) -> (element #1=w315:i32, element #2=w319:i32)  [unwired: 2 in]
                        n78 = Initialize Array(sgl nan ("element"), w315, w319) -> (w317:sgl[][])
                      }
                      frame True {
                        # "reset trigger count"
                        # "Trigger Found.  Retreive\npre-trigger data and append\nto remaining data from the \nDAQ buffer."
                        n79 = Increment(x=w325) -> (x+1=w324:i32)
                        n80 = call "Pretrigger Buffer (by ref).vi"("Mode"=enum16{"Initialize", "Add", "Read"}."Read") -> ("Pretrigger Data"=w334:sgl[][])  [unwired: 8 in, 1 out]
                        n81 = Array Subset(array=w336, index (row)=w324) -> (w335:sgl[][])  [unwired: 3 in]
                        n82 = Transpose 2D Array(2D array=w334) -> (transposed array=w328:sgl[][])
                        n83 = Array Size(array=w328) -> (size(s)=w327:i32[])
                        n84 = flat-sequence {
                          tunnel: w328 -> [_]
                          tunnel: w330 -> [w339]
                          tunnel: w329 -> [w338]
                          frame #0 {
                            n85 = call "Pretrigger Buffer (by ref).vi"("Mode"=enum16{"Initialize", "Add", "Read"}."Initialize", "Pretrigger Length"=w339, "# Channels"=w338) -> ()  [unwired: 6 in, 2 out]
                          }
                        }
                        n86 = Build Array (concatenate)(w328, w335) -> (w332:sgl[][])
                        n87 = Index Array(array=w327) -> (element=w326:i32)  [unwired: 1 in]
                        n88 = call "Trigger count.vi"("reset"=TRUE) -> ()  [unwired: 10 in, 1 out]
                        n89 = Decrement(x=w326) -> (x-1=w323:i32)
                      }
                    }
                  }
                  frame True {
                    # "Analog trigger has\nbeen activated"
                    # "Trigger is active.  Add all trigger data to the data buffer.  After adding data, check the size of the data buffer.\nIf the value is larger than the preset number of sample, remove the unnecessary samples."
                    n90 = Equal To 0?(x=w357) -> (x = 0?=w350:bool)
                    n91 = call "Organize Data With Analog Trigger.vi"("Coefficients"=w344, "Trigger Data Index"=w342, "System Type"=w341, "DAQ"=w365, "Channel Filter"=w359, "Sensor (scaling)"=w358) -> ("Scaled Data"=w360:sgl[][], "trigger data"=w355:sgl[])  [unwired: 8 in]
                    n92 = Transpose 2D Array(2D array=w360) -> (transposed array=w349:sgl[][])
                    n93 = Greater Or Equal?(x=w355, y=w354) -> (x >= y?=w353:bool[])
                    n94 = Or Array Elements(Boolean array=w353) -> (logical OR=w352:bool)
                    n95 = Array Size(array=w349) -> (size(s)=w364:i32[])
                    n96 = Not(x=w352) -> (.not. x?=w351:bool)
                    n97 = Index Array(array=w364, index=0) -> (element=w348:i32)
                    n98 = call "Trigger count.vi"("reset"=FALSE, "total to read"=w346, "# read"=w348) -> ("done?"=w345:bool)  [unwired: 8 in]
                    n99 = Select(t=w345, s=w350, f=w351) -> (s? t:f=w356:bool)
                    n100 = case shown="True" w356 {
                      tunnel: w349 -> [w370 w380]
                      tunnel: w346 -> [w369 _]
                      tunnel: [w368 w380] -> w362
                      tunnel: [FALSE TRUE] -> w361
                      tunnel: w350 -> [_ _]
                      tunnel: [0 0] -> w343
                      frame True {
                        # "All samples have been acquired.\nTrim off any extra samples\nand set DAQ to inactive state."
                        n101 = case shown="True" TRUE {
                          tunnel: w370 -> [w374 w378]
                          tunnel: [w373 w377] -> w368
                          tunnel: w369 -> [_ w375]
                          frame False {
                            n102 = Array Subset(array=w374, index (row)=0 ("index")) -> (w373:sgl[][])  [unwired: 3 in]
                          }
                          frame True {
                            n103 = Array Subset(array=w378, index (row)=0 ("index"), length (row)=w375) -> (w377:sgl[][])  [unwired: 2 in]
                          }
                        }
                      }
                      frame False {
                        # "Trigger is not complete.\nStore acquired data."
                      }
                    }
                  }
                }
              }
              frame "Analog Falling" {
                n104 = case shown="True" w397 {
                  tunnel: w396 -> [w415 w478]
                  tunnel: w395 -> [w414 w464]
                  tunnel: [w406 w474] -> w394
                  tunnel: [w407 w475] -> w393
                  tunnel: w392 -> [w410 w472]
                  tunnel: w391 -> [_ w460]
                  tunnel: w390 -> [w409 w471]
                  tunnel: w389 -> [_ w467]
                  tunnel: w388 -> [w403 w457]
                  tunnel: w387 -> [w402 _]
                  tunnel: w386 -> [w401 _]
                  tunnel: [w400 w456] -> w385
                  tunnel: w383 -> [w399 w455]
                  tunnel: w382 -> [w398 w454]
                  frame False {
                    # "Keep checking for analog\ntrigger."
                    # "No trigger is active.  Acquire data and process through the pretrigger sample buffer."
                    n105 = call "Organize Data With Analog Trigger.vi"("Coefficients"=w403, "Trigger Data Index"=w399, "System Type"=w398, "DAQ"=w415, "Channel Filter"=w410, "Sensor (scaling)"=w409) -> ("Scaled Data"=w411:sgl[][], "trigger data"=w413:sgl[])  [unwired: 8 in]
                    n106 = Transpose 2D Array(2D array=w411) -> (transposed array=w408:sgl[][])
                    n107 = Array Size(array=w413) -> (size(s)=w412:i32)
                    n108 = while {
                      tunnel: w408 -> [w441] mode=indexing
                      tunnel: w413 -> [w448] mode=indexing
                      tunnel: w414 -> [w446]
                      tunnel: [w444] -> w404
                      tunnel: w412 -> [w450]
                      tunnel: [w449] -> w405
                      i -> [w449]
                      stop <- w451 stop-if-true
                      w443 = u16 0 items=["Falling Edge", "Rising Edge"] ("slope")
                      w445 = u16 0 items=["Index", "Time"] ("mode")
                      n109 = Build Array(w448) -> (w447:sgl[])
                      n110 = Decrement(x=w450) -> (x-1=w452:i32)
                      n111 = call-poly <vilib>:"Basic Level Trigger Detection (obs).vi"("signal in"=w447, "level"=w446, "location mode"=w445, "trigger slope"=w443) -> ("trigger detected?"=w444:bool)  [unwired: 9 in, 2 out]
                      n112 = call "Pretrigger Buffer (by ref).vi"("Mode"=enum16{"Initialize", "Add", "Read"}."Add", "New Data"=w441) -> ()  [unwired: 7 in, 2 out]
                      n113 = Greater Or Equal?(x=w449, y=w452) -> (x >= y?=w442:bool)
                      n114 = Or(x=w444, y=w442) -> (x .or. y?=w451:bool)
                    }
                    n115 = case shown="True" w404 {
                      tunnel: [FALSE TRUE] -> w406
                      tunnel: w408 -> [w418 w436]
                      tunnel: [w417 w430] -> w407
                      tunnel: w405 -> [_ w431]
                      tunnel: w402 -> [_ w426]
                      tunnel: w401 -> [_ w425]
                      tunnel: [0 w424] -> w400
                      frame False {
                        (unwired) sgl[][] []
                        # "No trigger detected.  Keep on\ntrucking."
                        n116 = Array Size(array=w418) -> (size(s)=w422:i32[])
                        n117 = Index Array(array=w422) -> (element #1=w421:i32, element #2=w420:i32)  [unwired: 2 in]
                        n118 = Initialize Array(sgl nan ("element"), w421, w420) -> (w417:sgl[][])
                      }
                      frame True {
                        # "reset trigger count"
                        # "Trigger Found.  Retreive\npre-trigger data and append\nto remaining data from the \nDAQ buffer."
                        n119 = Increment(x=w431) -> (x+1=w432:i32)
                        n120 = call "Pretrigger Buffer (by ref).vi"("Mode"=enum16{"Initialize", "Add", "Read"}."Read") -> ("Pretrigger Data"=w434:sgl[][])  [unwired: 8 in, 1 out]
                        n121 = Array Subset(array=w436, index (row)=w432) -> (w435:sgl[][])  [unwired: 3 in]
                        n122 = Transpose 2D Array(2D array=w434) -> (transposed array=w427:sgl[][])
                        n123 = flat-sequence {
                          tunnel: w426 -> [w439]
                          tunnel: w425 -> [w438]
                          tunnel: w427 -> [_]
                          frame #0 {
                            n124 = call "Pretrigger Buffer (by ref).vi"("Mode"=enum16{"Initialize", "Add", "Read"}."Initialize", "Pretrigger Length"=w439, "# Channels"=w438) -> ()  [unwired: 6 in, 2 out]
                          }
                        }
                        n125 = Array Size(array=w427) -> (size(s)=w428:i32[])
                        n126 = Build Array (concatenate)(w427, w435) -> (w430:sgl[][])
                        n127 = Index Array(array=w428) -> (element=w424:i32)  [unwired: 1 in]
                        n128 = call "Trigger count.vi"("reset"=TRUE) -> ()  [unwired: 10 in, 1 out]
                      }
                    }
                  }
                  frame True {
                    # "Analog trigger has\nbeen activated"
                    # "Trigger is active.  Add all trigger data to the data buffer.  After adding data, check the size of the data buffer.\nIf the value is larger than the preset number of sample, remove the unnecessary samples."
                    n129 = Equal To 0?(x=w467) -> (x = 0?=w463:bool)
                    n130 = call "Organize Data With Analog Trigger.vi"("Coefficients"=w457, "Trigger Data Index"=w455, "System Type"=w454, "DAQ"=w478, "Channel Filter"=w472, "Sensor (scaling)"=w471) -> ("Scaled Data"=w473:sgl[][], "trigger data"=w470:sgl[])  [unwired: 8 in]
                    n131 = Transpose 2D Array(2D array=w473) -> (transposed array=w462:sgl[][])
                    n132 = Less Or Equal?(x=w470, y=w464) -> (x <= y?=w469:bool[])
                    n133 = Or Array Elements(Boolean array=w469) -> (logical OR=w468:bool)
                    n134 = Array Size(array=w462) -> (size(s)=w477:i32[])
                    n135 = Not(x=w468) -> (.not. x?=w465:bool)
                    n136 = Index Array(array=w477, index=0) -> (element=w461:i32)
                    n137 = call "Trigger count.vi"("reset"=FALSE, "total to read"=w460, "# read"=w461) -> ("done?"=w459:bool)  [unwired: 8 in]
                    n138 = Select(t=w459, s=w463, f=w465) -> (s? t:f=w466:bool)
                    n139 = case shown="True" w466 {
                      tunnel: w462 -> [w484 w493]
                      tunnel: w460 -> [w482 _]
                      tunnel: [w481 w493] -> w475
                      tunnel: [FALSE TRUE] -> w474
                      tunnel: w463 -> [_ _]
                      tunnel: [0 0] -> w456
                      frame True {
                        # "All samples have been acquired.\nTrim off any extra samples\nand set DAQ to inactive state."
                        n140 = case shown="True" TRUE {
                          tunnel: w484 -> [w487 w491]
                          tunnel: [w486 w490] -> w481
                          tunnel: w482 -> [_ w488]
                          frame False {
                            n141 = Array Subset(array=w487, index (row)=0 ("index")) -> (w486:sgl[][])  [unwired: 3 in]
                          }
                          frame True {
                            n142 = Array Subset(array=w491, index (row)=0 ("index"), length (row)=w488) -> (w490:sgl[][])  [unwired: 2 in]
                          }
                        }
                      }
                      frame False {
                        # "Trigger is not complete.\nStore acquired data."
                      }
                    }
                  }
                }
              }
            }
          }
        }
      }
      frame "Clear" {
        w501 = sgl[][] [] ("Scaled Data")
        # "Clear AI Task ID"
        n143 = call <vilib>:"DAQmx Clear Task.vi"("task in"=w505) -> ()  [unwired: 14 in, 1 out]
        n144 = call <vilib>:"DAQmx Clear Task.vi"("task in"=w499) -> ()  [unwired: 14 in, 1 out]
        n145 = call <vilib>:"DAQmx Clear Task.vi"("task in"=w497) -> ()  [unwired: 14 in, 1 out]
      }
    }
    n146 = Compound Arithmetic op=AND(w30, invert w32) -> (w31:bool)
    n147 = Transpose 2D Array(2D array=w17) -> (transposed array=w26:sgl[][])
    n148 = call "Realtime Data (by ref).vi"("New Data"=w26, "Enum"=enum16{"Init", "Read", "Write"}."Write") -> ()  [unwired: 1 out]
  }
  "error out" <- w8
  "Acquiring Data" <- w7
  "DAQ Complete Trigger" <- w6
  "Data" <- w3
  "Input Task OUT" <- w5
  "Pretrigger Size" <- w4
  "Ctr Task OUT" <- w2
  "DI Task OUT" <- w1
